vi "Update Values Buffer.vi"(7 "byte order (little-endian)":T1=enum."little-endian", 8 "error in (no error)":errorcluster, 9 "buffer data":T2={"decimation"=0, "avg bandwidth"=0.0, "channels"=[], "byte order"=enum."little-endian", "buffer descriptor"={"buffer type"=enum."Engine", "plugin id"=0, "group id"=0, "transfer id"=0, "offset"=0, "length"=0}, "values channels"={"index"=0, "count"=0, "engine offset"=0}, "select start offset"=18446744073709551615, "select end offset"=0, "channel index"=-1} {"channels"."configuration"."string offset" format="%d bytes"; "avg bandwidth" format="%.0g bytes"}, 10 "buffer in":u8[](array[numeric]), 11 "values buffer in":u8[](array[numeric])) -> (0 "error out":errorcluster, 2 "buffer out":u8[](array[numeric]), 3 "values buffer out":u8[](array[numeric]))   [LabVIEW 2017, in "DSF Core.lvlib"]
uses:
  DSF Core.lvlib
  Buffer Reader/Buffer Data.ctl
  Classes/Configuration/Core/Transfer/Channel Configuration.ctl
  Typedefs/Core Channel Configuration.ctl
  Typedefs/DSF Data Type.ctl
  Typedefs/DSF Settings Info.ctl
  Typedefs/DSF Byte Order.ctl
  Classes/Thread/Data Server/DSF Buffer Subset Descriptor.ctl
  Typedefs/DSF Buffer Type.ctl
  Values Channels.ctl
  Classes/Framework/Framework.lvclass
  Classes/Configuration/Core/Channel/Channel Configuration.lvclass
  Classes/Configuration/Core/Transfer/Transfer Configuration.lvclass
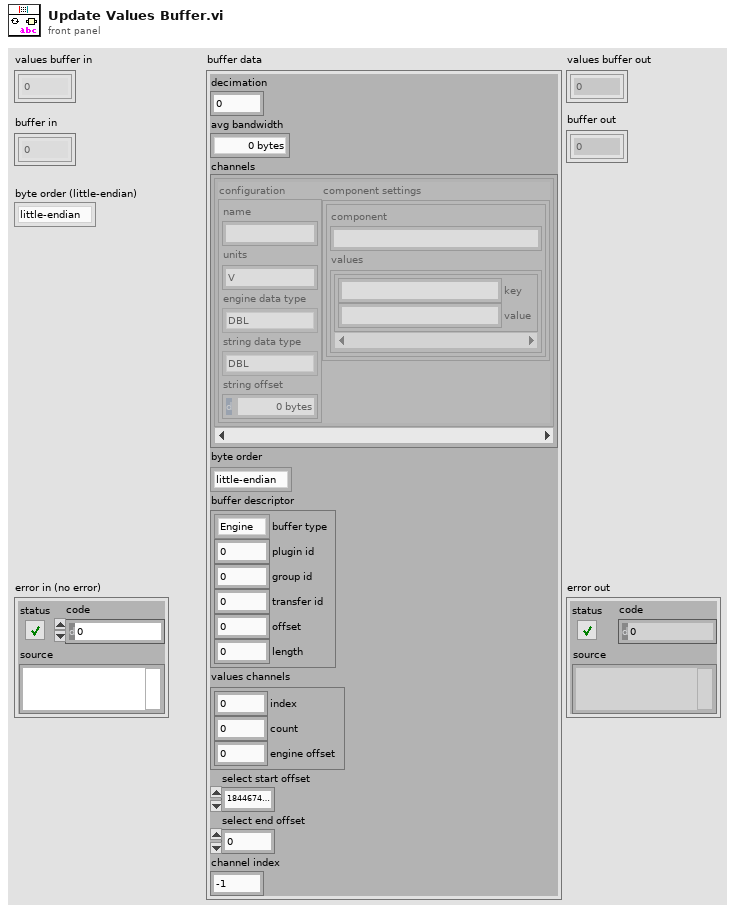
[diagram p1: front panel]
types:
  T1 = typedef "DSF Core.lvlib/DSF Byte Order.ctl" = enum8{"big-endian", "little-endian"}
  T2 = typedef "DSF Core.lvlib/Buffer Data.ctl" = cluster{"decimation":u64, "avg bandwidth":dbl, "channels":T3[], "byte order":T1, "buffer descriptor":T7, "values channels":T9, "select start offset":u64, "select end offset":u64, "channel index":i32}
  T3 = typedef "DSF Core.lvlib/Transfer Configuration.lvclass/Channel Configuration.ctl" = cluster{"configuration":T4, "component settings":T6[]}
  T4 = typedef "DSF Core.lvlib/Channel Configuration.lvclass/Core Channel Configuration.ctl" = cluster{"name":string, "units":string, "engine data type":T5, "string data type":T5, "string offset":u64}
  T5 = typedef "DSF Core.lvlib/DSF Data Type.ctl" = enum8{"Bool", "SGL", "DBL", "I8", "I16", "I32", "I64", "U8", "U16", "U32", "U64"}
  T6 = typedef "DSF Core.lvlib/DSF Settings Info.ctl" = cluster{"component":string, "values":cluster{"key":string, "value":string}[]}
  T7 = typedef "DSF Core.lvlib/DSF Buffer Subset Descriptor.ctl" = cluster{"buffer type":T8, "plugin id":i32, "group id":i32, "transfer id":i32, "offset":u64, "length":i64}
  T8 = typedef "DSF Core.lvlib/DSF Buffer Type.ctl" = enum16{"Engine", "String"}
  T9 = typedef "DSF Core.lvlib/Values Channels.ctl" = cluster{"index":i32, "count":i32, "engine offset":u64}
  T10 = enum16{"big-endian, network order", "native, host order", "little-endian"}
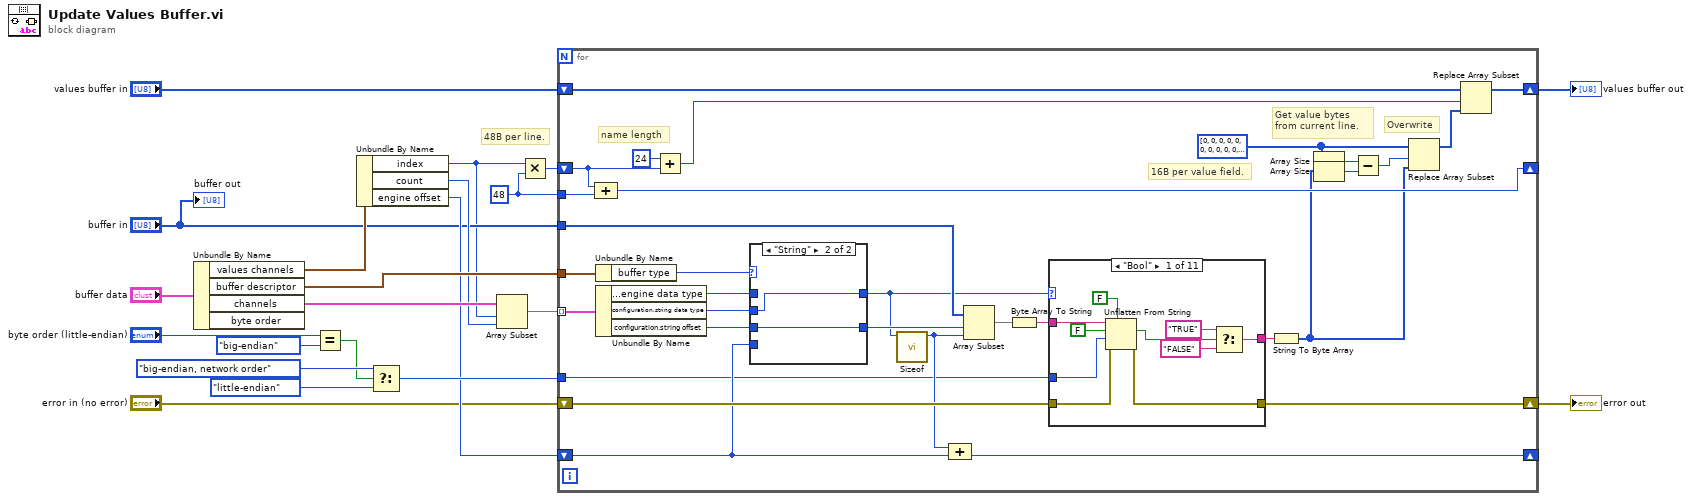
[diagram p0: block diagram]
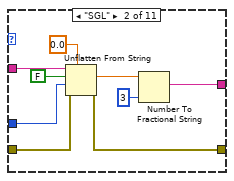
[diagram p3: hidden frame]
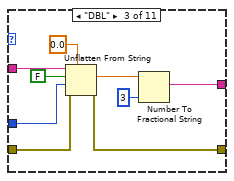
[diagram p4: hidden frame]
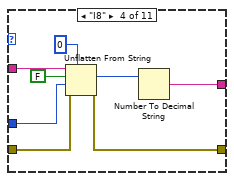
[diagram p5: hidden frame]
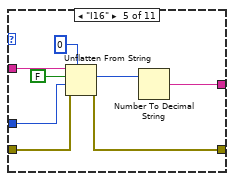
[diagram p6: hidden frame]
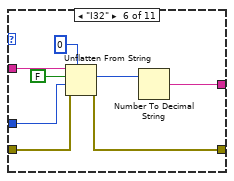
[diagram p7: hidden frame]
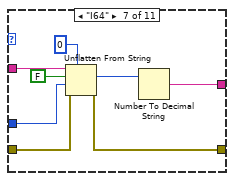
[diagram p8: hidden frame]
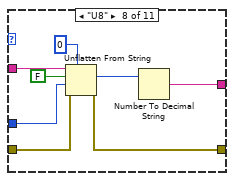
[diagram p9: hidden frame]
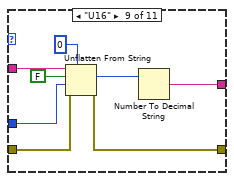
[diagram p10: hidden frame]
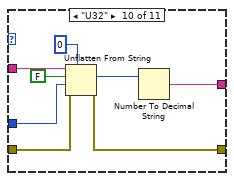
[diagram p11: hidden frame]
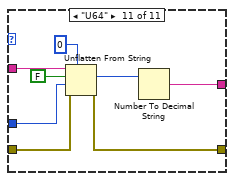
[diagram p12: hidden frame]
diagram:
  w2 = 48 ("x")
  # "48B per line."
  n1 = Unbundle By Name("buffer data") -> ("values channels"=w19:T9, "buffer descriptor"=w18:T7, "channels"=w17:T3[])  [unwired: 1 out]
  n2 = Equal?(x="byte order (little-endian)", y=DSF_Byte_Order."big-endian") -> (x = y?=w6:bool)
  n3 = Unbundle By Name(w19) -> ("index"=w3:i32, "count"=w10:i32, "engine offset"=w8:u64)
  n4 = Select(t=T10."big-endian, network order" ("byte order (0:big-endian, network order)"), s=w6, f=T10."little-endian") -> (s? t:f=w13:T10)
  n5 = Array Subset(array=w17, index=w3, length=w10) -> (w21:T3[])
  n6 = Multiply(x=w3, y=w2) -> (x*y=w4:i32)
  n7 = for {
    shift-right: [w30] -> w9
    shift-left: "error in (no error)" -> [w52]
    tunnel: w21 -> [w51] mode=indexing
    tunnel: w18 -> [w45]
    shift-right: [w46] -> _
    shift-left: w8 -> [w44]
    tunnel: w13 -> [w39]
    shift-right: [w42] -> w11
    shift-left: "values buffer in" -> [w43]
    tunnel: "buffer in" -> [w38]
    shift-right: [w31] -> _
    shift-left: w4 -> [w32]
    tunnel: w2 -> [w33]
    w22 = u8[] [0, 0, 0, 0, 0, 0, 0, 0, 0, 0, 0, 0, 0, 0, 0, 0]
    # "16B per value field."
    # "name length"
    # "Overwrite"
    # "Get value bytes from current line."
    n8 = Compound Arithmetic op=ADD(w32, w33) -> (w31:i32)
    n9 = Unbundle By Name(w45) -> ("buffer type"=w27:T8)
    n10 = Unbundle By Name(w51) -> ("configuration.engine data type"=w48:T5, "configuration.string data type"=w49:T5, "configuration.string offset"=w50:u64)
    n11 = Add(x=24, y=w32) -> (x+y=w40:i32)
    n12 = case shown="\"String\"" w27 {
      tunnel: w50 -> [_ w56]
      tunnel: [w53 w56] -> w29
      tunnel: w49 -> [_ w55]
      tunnel: w48 -> [w54 _]
      tunnel: w44 -> [w53 _]
      tunnel: [w54 w55] -> w28
      frame "Engine" {
      }
      frame "String" {
      }
    }
    n13 = call "Sizeof.vi"("data type"=w28) -> ("size in bytes"=w47:u64)  [unwired: 9 in, 1 out]
    n14 = Compound Arithmetic op=ADD(w47, w44) -> (w46:u64)
    n15 = Array Subset(array=w38, index=w29, length=w47) -> (w26:u8[])
    n16 = Byte Array To String(unsigned byte array=w26) -> (string=w25:string)
    n17 = case shown="\"Bool\"" w28 {
      tunnel: w52 -> [w66 w75 w84 w92 w100 w108 w116 w124 w132 w140 w148]
      tunnel: [w65 w74 w83 w91 w99 w107 w115 w123 w131 w139 w147] -> w30
      tunnel: w39 -> [w60 w71 w80 w88 w96 w104 w112 w120 w128 w136 w144]
      tunnel: [w59 w68 w77 w86 w94 w101 w110 w118 w126 w134 w142] -> w23
      tunnel: w25 -> [w57 w67 w76 w85 w93 w102 w109 w117 w125 w133 w141]
      frame "Bool" {
        n18 = Unflatten From String(type=FALSE, binary string=w57, data includes array or string size? (T)=FALSE, byte order (0:big-endian, network order)=w60, error in (no error)=w66) -> (value=w58:bool, error out=w65:errorcluster)  [unwired: 1 out]
        n19 = Select(t="TRUE", s=w58, f="FALSE") -> (s? t:f=w59:string)
      }
      frame "SGL" {
        n20 = Unflatten From String(type=sgl 0.0, binary string=w67, data includes array or string size? (T)=FALSE, byte order (0:big-endian, network order)=w71, error in (no error)=w75) -> (value=w69:sgl, error out=w74:errorcluster)  [unwired: 1 out]
        n21 = Number To Fractional String(number=w69, precision (6)=i16 3) -> (F-format string=w68:string)  [unwired: 2 in]
      }
      frame "DBL" {
        n22 = Unflatten From String(type=0.0, binary string=w76, data includes array or string size? (T)=FALSE, byte order (0:big-endian, network order)=w80, error in (no error)=w84) -> (value=w78:dbl, error out=w83:errorcluster)  [unwired: 1 out]
        n23 = Number To Fractional String(number=w78, precision (6)=i16 3) -> (F-format string=w77:string)  [unwired: 2 in]
      }
      frame "I8" {
        n24 = Unflatten From String(type=i8 0, binary string=w85, data includes array or string size? (T)=FALSE, byte order (0:big-endian, network order)=w88, error in (no error)=w92) -> (value=w87:i8, error out=w91:errorcluster)  [unwired: 1 out]
        n25 = Number To Decimal String(number=w87) -> (decimal integer string=w86:string)  [unwired: 1 in]
      }
      frame "I16" {
        n26 = Unflatten From String(type=i16 0, binary string=w93, data includes array or string size? (T)=FALSE, byte order (0:big-endian, network order)=w96, error in (no error)=w100) -> (value=w95:i16, error out=w99:errorcluster)  [unwired: 1 out]
        n27 = Number To Decimal String(number=w95) -> (decimal integer string=w94:string)  [unwired: 1 in]
      }
      frame "I32" {
        n28 = Unflatten From String(type=0, binary string=w102, data includes array or string size? (T)=FALSE, byte order (0:big-endian, network order)=w104, error in (no error)=w108) -> (value=w103:i32, error out=w107:errorcluster)  [unwired: 1 out]
        n29 = Number To Decimal String(number=w103) -> (decimal integer string=w101:string)  [unwired: 1 in]
      }
      frame "I64" {
        n30 = Unflatten From String(type=i64 0, binary string=w109, data includes array or string size? (T)=FALSE, byte order (0:big-endian, network order)=w112, error in (no error)=w116) -> (value=w111:i64, error out=w115:errorcluster)  [unwired: 1 out]
        n31 = Number To Decimal String(number=w111) -> (decimal integer string=w110:string)  [unwired: 1 in]
      }
      frame "U8" {
        n32 = Unflatten From String(type=u8 0, binary string=w117, data includes array or string size? (T)=FALSE, byte order (0:big-endian, network order)=w120, error in (no error)=w124) -> (value=w119:u8, error out=w123:errorcluster)  [unwired: 1 out]
        n33 = Number To Decimal String(number=w119) -> (decimal integer string=w118:string)  [unwired: 1 in]
      }
      frame "U16" {
        n34 = Unflatten From String(type=u16 0, binary string=w125, data includes array or string size? (T)=FALSE, byte order (0:big-endian, network order)=w128, error in (no error)=w132) -> (value=w127:u16, error out=w131:errorcluster)  [unwired: 1 out]
        n35 = Number To Decimal String(number=w127) -> (decimal integer string=w126:string)  [unwired: 1 in]
      }
      frame "U32" {
        n36 = Unflatten From String(type=u32 0, binary string=w133, data includes array or string size? (T)=FALSE, byte order (0:big-endian, network order)=w136, error in (no error)=w140) -> (value=w135:u32, error out=w139:errorcluster)  [unwired: 1 out]
        n37 = Number To Decimal String(number=w135) -> (decimal integer string=w134:string)  [unwired: 1 in]
      }
      frame "U64" {
        n38 = Unflatten From String(type=u64 0, binary string=w141, data includes array or string size? (T)=FALSE, byte order (0:big-endian, network order)=w144, error in (no error)=w148) -> (value=w143:u64, error out=w147:errorcluster)  [unwired: 1 out]
        n39 = Number To Decimal String(number=w143) -> (decimal integer string=w142:string)  [unwired: 1 in]
      }
    }
    n40 = String To Byte Array(string=w23) -> (unsigned byte array=w24:u8[])
    n41 = Array Size(array=w22) -> (size(s)=w37:i32)
    n42 = Array Size(array=w24) -> (size(s)=w36:i32)
    n43 = Subtract(x=w37, y=w36) -> (x-y=w35:i32)
    n44 = Replace Array Subset(array=w22, new element=w24, index=w35) -> (w34:u8[])
    n45 = Replace Array Subset(array=w43, new element=w34, index=w40) -> (w42:u8[])
  }
  "values buffer out" <- w11
  "error out" <- w9
  "buffer out" <- "buffer in"
